vi "Find_VISA.vi"() -> (0 "错误输出":errorcluster, 1 "虚拟放射源VISA":string, 2 "多道VISA":string)   [LabVIEW 2014]
panel:
  out "返回数":u32
  out "查找列表":string[](array[string])
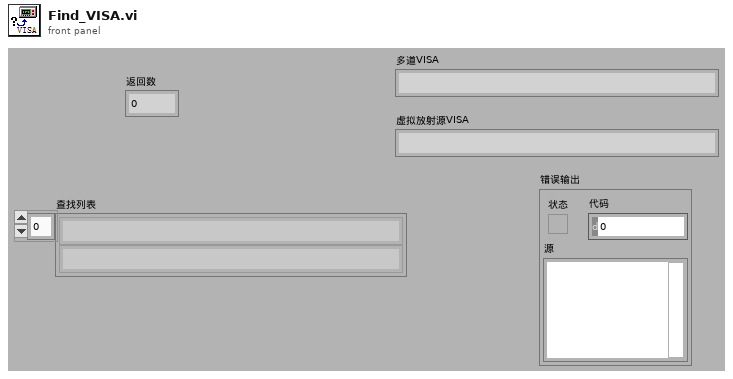
[diagram p1: front panel]
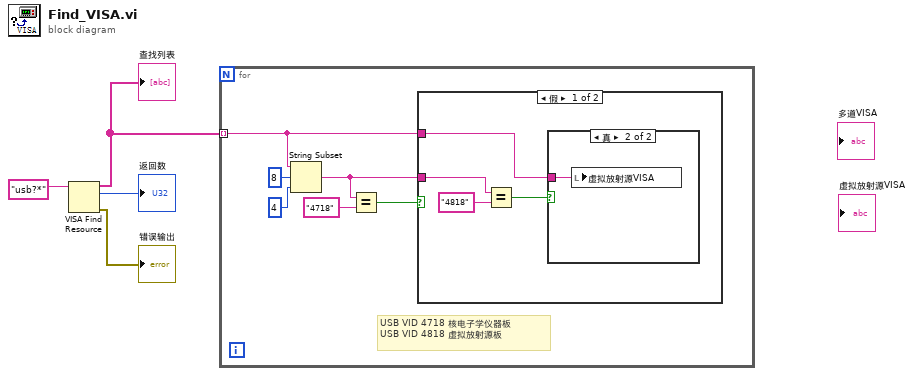
[diagram p0: block diagram]
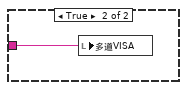
[diagram p3: hidden frame]
diagram:
  n1 = VISA Find Resource(11:"usb?*" ("表达式(\"?*\")")) -> (0:→"错误输出":errorcluster, 2:→"返回数":u32, 3:w2:string[])  [unwired: 2 in]
  "查找列表" <- w2
  n2 = for {
    tunnel: w2 -> [w6] mode=indexing
    # "USB VID 4718 核电子学仪器板\nUSB VID 4818 虚拟放射源板"
    n3 = String Subset(string=w6, offset (0)=8 ("偏移量(0)"), length (rest)=4 ("长度（剩余）")) -> (substring=w5:string)
    n4 = Equal?(x=w5, y="4718") -> (x = y?=w7:bool)
    n5 = case shown="假" w7 {
      tunnel: w6 -> [w11 w16]
      tunnel: w5 -> [w12 _]
      frame False {
        n6 = Equal?(x=w12, y="4818") -> (x = y?=w13:bool)
        n7 = case shown="真" w13 {
          tunnel: w11 -> [_ w15]
          frame False {
          }
          frame True {
            n8 = local write "虚拟放射源VISA"(w15) -> ()
          }
        }
      }
      frame True {
        n9 = local write "多道VISA"(w16) -> ()
      }
    }
  }
